vi "Get_Available_Cameras.vi"() -> (0 "error out":errorcluster, 1 "Cameras":string[](array[string]))   [LabVIEW 2020]
doc: "Self-test all hardware devices on the system specified."
panel:
  in  "User Name":string
  in  "Password":string
  in  "Target (localhost)":refnum<k21>="localhost"
  # "Remote call to remove IMAQ library-requiring VIs from the BD"
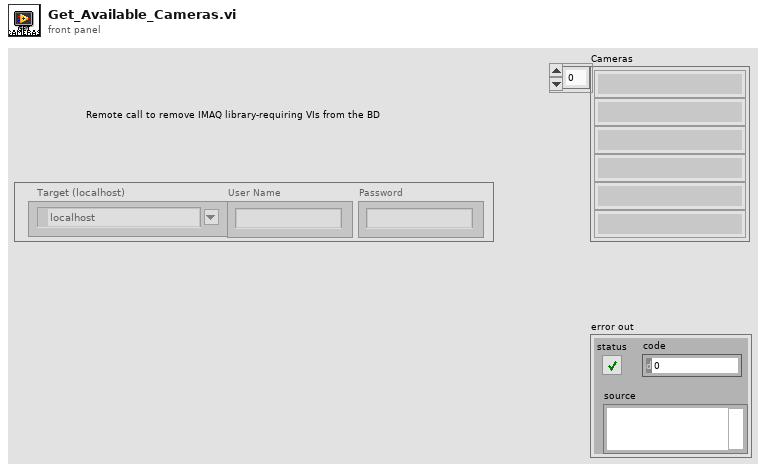
[diagram p1: front panel]
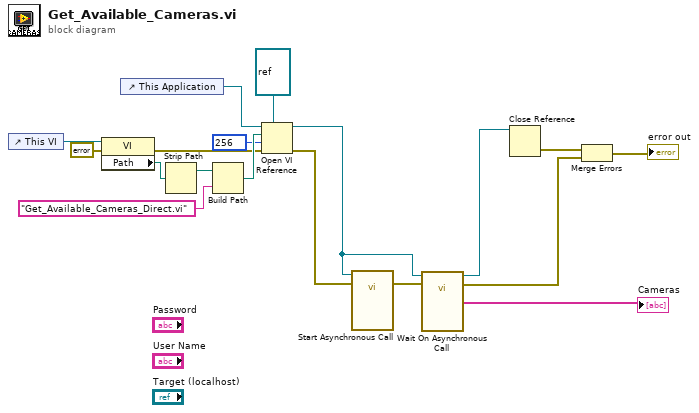
[diagram p0: block diagram]
diagram:
  n1 = control-ref of="This VI"() -> (w12:refnum<vi>)
  n2 = property class="VI"(reference=w12, error in=errorcluster {"status"=FALSE, "code"=0, "source"=""} ("error in (no error)")) -> (error out=w9:errorcluster, "Path"=w5:path)  [unwired: 1 out]
  n3 = control-ref of="This Application"() -> (w7:refnum<vi>)
  n4 = Strip Path(path=w5) -> (stripped path=w4:path)  [unwired: 1 out]
  n5 = Build Path(base path=w4, name or relative path="Get_Available_Cameras_Direct.vi") -> (appended path=w10:path)
  n6 = Open VI Reference(type specifier VI Refnum (for type only)=refnum<vi> refnum, application reference (local)=w7, vi path=w10, options=256, error in (no error)=w9) -> (vi reference=w18:refnum<vi>, error out=w3:errorcluster)  [unwired: 1 in]
  n7 = call-by-ref "Start Asynchronous Call"(reference=w18, error in=w3) -> (error out=w17:errorcluster)  [unwired: 3 in, 2 out]
  n8 = call-by-ref "Wait On Asynchronous Call"(reference=w18, error in=w17) -> (reference out=w2:refnum<vi>, error out=w16:errorcluster, "Cameras"=→"Cameras":string[])  [unwired: 3 in]
  n9 = Close Reference(reference=w2) -> (error out=w14:errorcluster)  [unwired: 1 in]
  n10 = Merge Errors(w14, w16) -> (→"error out":errorcluster)
